vi "My Nonlinear Curve Fit LM bounds.vi"(0 "Y":dbl[](array[numeric]), 1 "f(x,a)":T4, 2 "data":variant, 5 "X":dbl[](array[numeric]), 7 "Weight":dbl[](array[numeric]), 9 "initial parameters":dbl[](array[numeric]), 11 "error in (no error)":errorcluster, 12 "termination":cluster{"max iteration":i32, "tolerance":dbl}={"max iteration"=200, "tolerance"=1e-08}, 13 "parameter bounds":T2, 14 "method":T3 items=["Least Square", "Least Absolute Residual", "Bisquare"]) -> (3 "Fit Aborted?":bool, 4 "best nonlinear fit":dbl[](array[numeric]), 6 "best fit parameters":dbl[](array[numeric]), 8 "covariance":T5, 10 "Fit Statistics":T1, 15 "error out":errorcluster)   [LabVIEW 2019]
uses:
  <vilib>/Analysis/Matrix/Datatypes/RealMatrix.ctl
  <vilib>/gmath/NumericalOptimization/LM model function reference.ctl
  <vilib>/Analysis/6fits.llb/Curve Fitting Criteria.ctl
  Fit Statistics.ctl
  My Fit Stopping Criteria.ctl
  <vilib>/gmath/NumericalOptimization/LM model function.ctl
  <vilib>/gmath/NumericalOptimization/LM_output select.ctl
  Abort Fit Global.vi
  <vilib>/gmath/NI_Gmath.lvlib
  <vilib>/Analysis/NI_AALBase.lvlib
  <vilib>/Analysis/Matrix/NI_Matrix.lvlib
  <vilib>/Analysis/NI_AALPro.lvlib
panel:
  out "Waveform Graph":dbl[](graph)
  in  "Delay (ms)":i32
  in  "Debug":bool
  out "Parameters Chart":dbl[][](graph)
  out "Function & Fit Graph":cluster{"New Coefficients":dbl[]}[](graph)
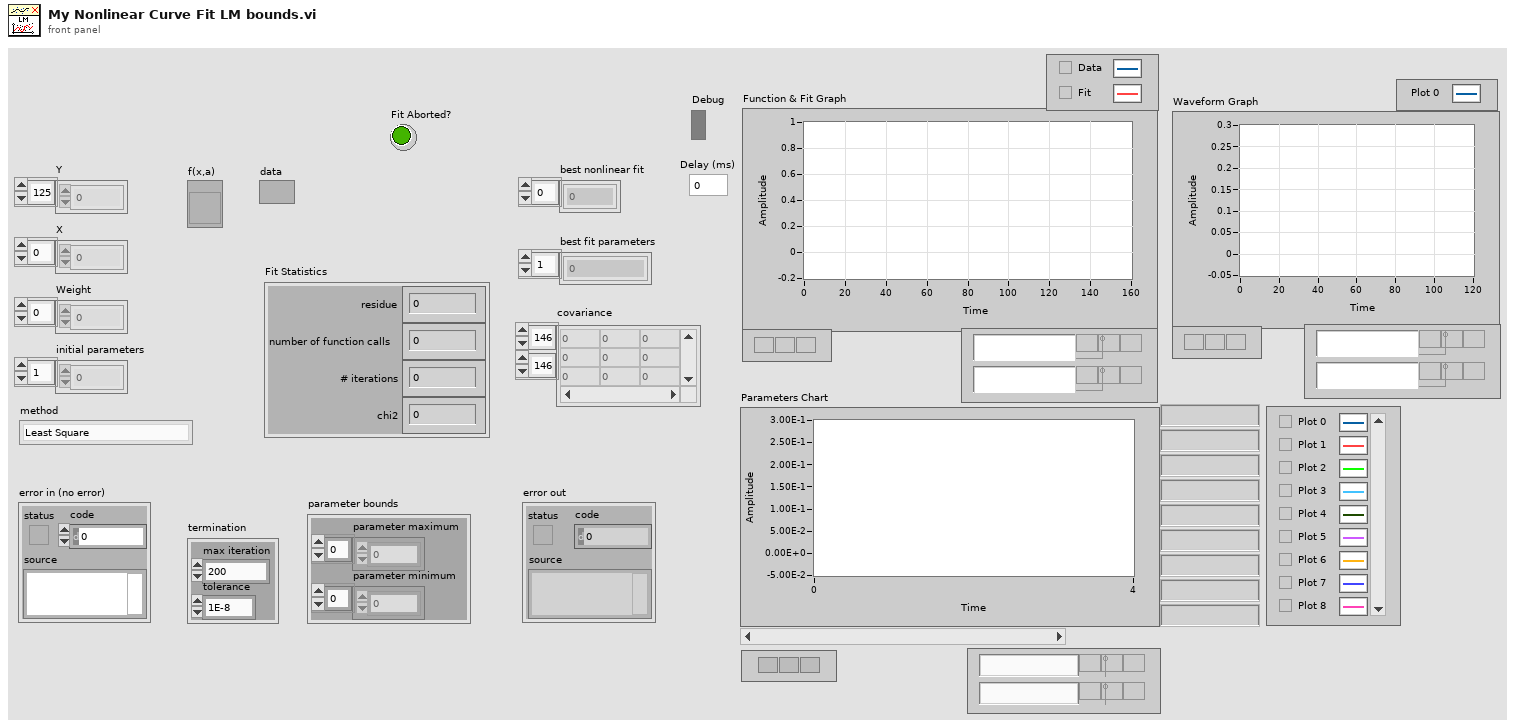
[diagram p1: front panel]
types:
  T1 = typedef "Fit Statistics.ctl" = cluster{"# iterations":i32, "number of function calls":i32, "chi2":dbl, "residue":dbl}
  T2 = cluster{"parameter minimum":dbl[], "parameter maximum":dbl[]}
  T3 = typedef "NI_AALPro.lvlib/Curve Fitting Criteria.ctl" = u16
  T4 = typedef "NI_Gmath.lvlib/LM model function reference.ctl" = refnum<vi>
  T5 = typedef "NI_Matrix.lvlib/RealMatrix.ctl" = dbl[][]
  T6 = typedef "NI_Gmath.lvlib/LM model function.ctl" = cluster{"f(x,a)":T4, "data":variant}
  T7 = typedef "My Fit Stopping Criteria.ctl" = cluster{"function tolerance":dbl, "parameter tolerance":dbl, "max iterations":i32, "max function calls":i32, "gradient tolerance":dbl, "max time (sec)":dbl, "initial tick count":u32, "min lambda":dbl, "max lambda":dbl}
  T8 = typedef "NI_Gmath.lvlib/LM_output select.ctl" = cluster{"model function":bool, "gradient":bool}
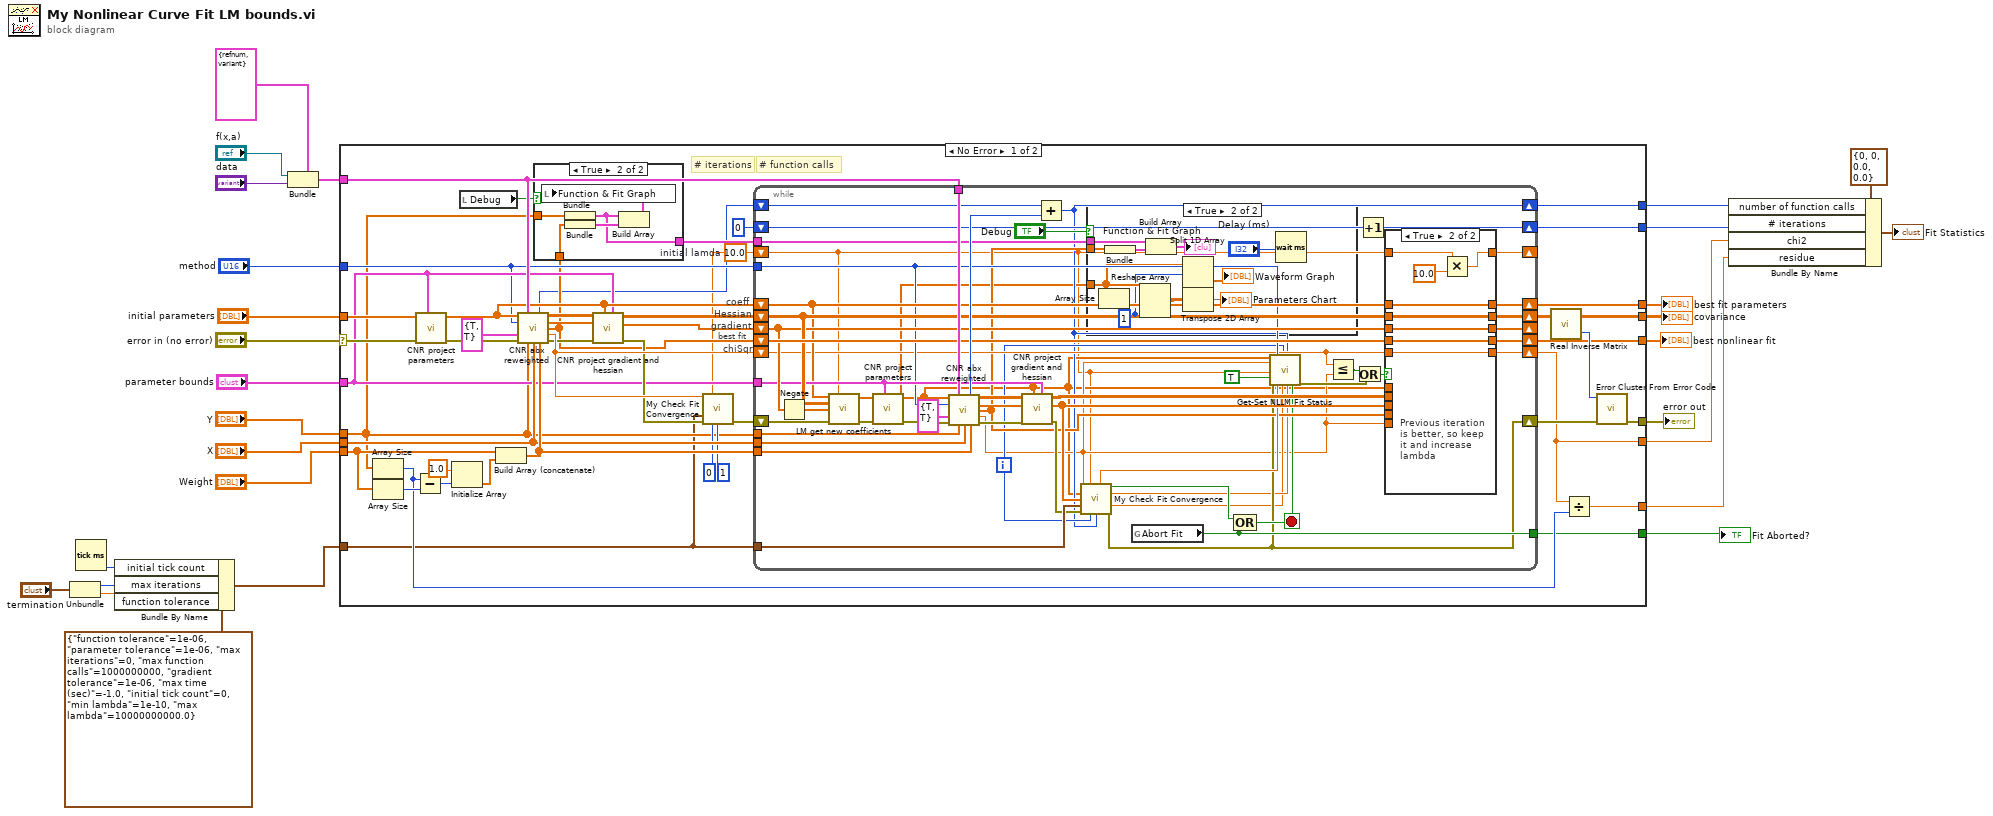
[diagram p0: block diagram]
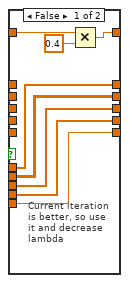
[diagram p4: hidden frame]
diagram:
  n1 = Unbundle("termination") -> ("max iteration"=w17:i32, "tolerance"=w16:dbl)
  n2 = Tick Count (ms)() -> (millisecond timer value=w2:u32)
  n3 = Bundle By Name(cluster=T7 {"function tolerance"=1e-06, "parameter tolerance"=1e-06, "max iterations"=0, "max function calls"=1000000000, "gradient tolerance"=1e-06, "max time (sec)"=-1.0, "initial tick count"=0, "min lambda"=1e-10, "max lambda"=10000000000.0} ("my stopping criteria"), "initial tick count"=w2, "max iterations"=w17, "function tolerance"=w16) -> (w1:T7)
  n4 = Bundle(cluster=T6 {"f(x,a)"=refnum, "data"=variant} ("model function"), "f(x,a)"="f(x,a)", "data"="data") -> (w13:T6)
  n5 = case shown="No Error" "error in (no error)" {
    selector: "error in (no error)" -> [w49 w160]
    tunnel: [w52 _] -> w28
    tunnel: [w73 _] -> w4
    tunnel: "initial parameters" -> [w50 _]
    tunnel: [w60 _] -> w26
    tunnel: [w71 _] -> w25
    tunnel: "Weight" -> [w67 _]
    tunnel: "Y" -> [w37 _]
    tunnel: w1 -> [w30 _]
    tunnel: "X" -> [w61 _]
    tunnel: [w65 w160] -> w21
    tunnel: w13 -> [w62 _]
    tunnel: [w54 _] -> w8
    tunnel: "method" -> [w39 _]
    tunnel: "parameter bounds" -> [w42 _]
    tunnel: [w38 _] -> w9
    tunnel: [w33 _] -> w5
    tunnel: [w31 _] -> w6
    frame No Error {
      w29 = 10.0  # initial lamda
      # "# iterations"
      # "# function calls"
      # "best fit"
      # "chiSqr"
      # "gradient"
      # "Hessian"
      # "coeff"
      n6 = Array Size(array=w37) -> (size(s)=w51:i32)
      n7 = Array Size(array=w67) -> (size(s)=w70:i32)
      n8 = Subtract(x=w51, y=w70) -> (x-y=w69:i32)
      n9 = call <vilib>:"CNR project parameters.vi"("bounds"=w42, "error in"=w49, "parameters"=w50) -> ("error out"=w48:errorcluster, "projected parameters"=w43:dbl[])  [unwired: 7 out]
      n10 = Initialize Array(1.0, w69) -> (w68:dbl[])
      n11 = local read "Debug"() -> (w34:bool)
      n12 = Build Array (concatenate)(w67, w68) -> (w74:dbl[])
      n13 = call <vilib>:"CNR abx reweighted.vi"("parameters"=w43, "model function"=w62, "method"=w39, "output control"=T8 {"model function"=TRUE, "gradient"=TRUE}, "error in (no error)"=w48, "Y"=w37, "X"=w61, "Weight"=w74) -> ("number of function calls"=w32:i32, "Hessian"=w45:T5, "gradient"=w44:dbl[], "best fit"=w35:dbl[], "chiSqr"=w64:dbl, "error out"=w47:errorcluster)  [unwired: 1 in, 1 out]
      n14 = case shown="True" w34 {
        tunnel: w37 -> [_ w79]
        tunnel: [_ w76] -> w36
        tunnel: w35 -> [_ w78]
        frame False {
        }
        frame True {
          n15 = Bundle("Y"=w79) -> (w76:cluster{"Y":dbl[]})  [unwired: 1 in]
          n16 = Bundle("best fit"=w78) -> (w77:cluster{"best fit":dbl[]})  [unwired: 1 in]
          n17 = Build Array(w76, w77) -> (w75:cluster{"best fit":dbl[]}[])
          n18 = local write "Function & Fit Graph"(w75) -> ()
        }
      }
      n19 = call <vilib>:"CNR project gradient and hessian.vi"("bounds"=w42, "projected parameters"=w43, "error in"=w47, "gradient"=w44, "Hessian"=w45) -> ("error out"=w46:errorcluster, "projected gradient"=w40:dbl[], "projected Hessian"=w41:T5)  [unwired: 1 in, 3 out]
      n20 = call "My Check Fit Convergence.vi"("Chi 2"=w64, "Lambda"=w29, "my stopping criteria"=w30, "Error In"=w46, "current iteration"=0, "number of function evaluations"=1) -> ("error out"=w63:errorcluster)  [unwired: 5 in, 4 out]
      n21 = while {
        tunnel: w61 -> [w127]
        tunnel: w37 -> [w95]
        tunnel: w74 -> [w126]
        shift-left: w64 -> [w99]
        shift-right: [w114] -> w33
        shift-left: w40 -> [w120]
        shift-right: [w130] -> _
        shift-left: w41 -> [w121]
        shift-right: [w131] -> w56
        shift-left: w43 -> [w101]
        shift-right: [w115] -> w52
        shift-left: w29 -> [w80]
        shift-right: [w128] -> _
        shift-right: [w86] -> w59
        shift-left: w63 -> [w129]
        tunnel: w62 -> [w125]
        tunnel: w30 -> [w117]
        shift-right: [w88] -> w54
        shift-left: w32 -> [w124]
        shift-right: [w122] -> w60
        shift-left: w35 -> [w123]
        shift-right: [w90] -> w31
        shift-left: 0 -> [w91]
        tunnel: w39 -> [w100]
        tunnel: w42 -> [w107]
        tunnel: [w102] -> w38
        tunnel: w36 -> [w94]
        i -> [w89]
        stop <- w87 stop-if-true
        n22 = Negate(x=w120) -> (-x=w103:dbl[])
        n23 = call <vilib>:"LM get new coefficients.vi"("Coefficients"=w101, "lamda"=w80, "Alpha"=w121, "Beta"=w103, "error in (no error)"=w129) -> ("New Coefficients"=w96:dbl[], "error out"=w113:errorcluster)  [unwired: 9 out]
        n24 = call <vilib>:"CNR project parameters.vi"("bounds"=w107, "error in"=w113, "parameters"=w96) -> ("error out"=w112:errorcluster, "projected parameters"=w81:dbl[])  [unwired: 7 out]
        n25 = call <vilib>:"CNR abx reweighted.vi"("parameters"=w81, "model function"=w125, "method"=w100, "output control"=T8 {"model function"=TRUE, "gradient"=TRUE}, "error in (no error)"=w112, "Y"=w95, "X"=w127, "Weight"=w126) -> ("number of function calls"=w132:i32, "Hessian"=w106:T5, "gradient"=w109:dbl[], "best fit"=w92:dbl[], "chiSqr"=w82:dbl, "error out"=w111:errorcluster)  [unwired: 1 in, 1 out]
        n26 = call <vilib>:"CNR project gradient and hessian.vi"("bounds"=w107, "projected parameters"=w81, "error in"=w111, "gradient"=w109, "Hessian"=w106) -> ("error out"=w110:errorcluster, "projected gradient"=w108:dbl[], "projected Hessian"=w105:T5)  [unwired: 1 in, 3 out]
        n27 = Add(x=w124, y=w132) -> (x+y=w88:i32)
        n28 = call "My Check Fit Convergence.vi"("Chi 2"=w82, "Lambda"=w80, "Parameters"=w81, "gradient"=w108, "my stopping criteria"=w117, "Error In"=w110, "current iteration"=w89, "number of function evaluations"=w88) -> ("|Delta Chi 2|/Chi 2"=w97:dbl, "stop?"=w116:bool, "|Delta Chi 2|"=w84:dbl, "Max |Delta a| /|a|"=w83:dbl, "error out"=w86:errorcluster)  [unwired: 3 in]
        n29 = case shown="True" "Debug" {
          tunnel: w81 -> [_ w135]
          tunnel: w94 -> [_ w143]
          tunnel: w92 -> [_ w140]
          frame False {
          }
          frame True {
            w133 = 1 ("dimension size")
            n30 = Array Size(array=w135) -> (size(s)=w139:i32)
            n31 = Bundle("best fit"=w140) -> (w142:cluster{"best fit":dbl[]})  [unwired: 1 in]
            n32 = Reshape Array(w135, w139, w133) -> (w138:dbl[][])
            n33 = Build Array(w143, w142) -> (→"Function & Fit Graph":cluster{"best fit":dbl[]}[])
            n34 = Split 1D Array(array=w135, index=w133) -> (second subarray=→"Waveform Graph":dbl[])  [unwired: 1 out]
            n35 = Transpose 2D Array(2D array=w138) -> (transposed array=→"Parameters Chart":dbl[][])
            n36 = Wait (ms)(milliseconds to wait="Delay (ms)") -> ()  [unwired: 1 out]
          }
        }
        n37 = global read "Abort Fit Global.vi" "Abort Fit"() -> (w102:bool)
        n38 = Compound Arithmetic op=OR(w116, w102) -> (w87:bool)
        n39 = call "Get-Set NLLM Fit Status.vi"("Fit Parameters"=w81, "chiSqr"=w82, "Lambda"=w80, "Get(F)/Set"=TRUE, "Error In"=w86, "method"=w100, "|Delta Chi 2|/Chi 2"=w97, "# Iterations"=w89, "Max |Delta a| /|a|"=w83, "# Function Calls"=w88, "|Delta Chi 2|"=w84, "Done"=w87) -> ("Error Out"=w85:errorcluster)  [unwired: 6 in, 1 out]
        n40 = Less Or Equal?(x=w99, y=w82) -> (x <= y?=w119:bool)
        n41 = Or(x=w119, y=w85) -> (x .or. y?=w118:bool)
        n42 = Increment(x=w91) -> (x+1=w90:i32)
        n43 = case shown="True" w118 {
          tunnel: [w150 w159] -> w131
          tunnel: w121 -> [_ w159]
          tunnel: [w149 w158] -> w130
          tunnel: w81 -> [w146 _]
          tunnel: w120 -> [_ w158]
          tunnel: w101 -> [_ w157]
          tunnel: [w146 w157] -> w115
          tunnel: [w151 w155] -> w128
          tunnel: w99 -> [_ w156]
          tunnel: w82 -> [w147 _]
          tunnel: [w147 w156] -> w114
          tunnel: w80 -> [w145 w153]
          tunnel: w105 -> [w150 _]
          tunnel: w108 -> [w149 _]
          tunnel: w123 -> [_ w154]
          tunnel: w92 -> [w148 _]
          tunnel: [w148 w154] -> w122
          frame False {
            # "Current iteration\nis better, so use\nit and decrease \nlambda"
            n44 = Multiply(x=w145, y=0.4) -> (x*y=w151:dbl)
          }
          frame True {
            # "Previous iteration\nis better, so keep\nit and increase \nlambda"
            n45 = Multiply(x=w153, y=10.0) -> (x*y=w155:dbl)
          }
        }
      }
      n46 = call <vilib>:"Real Inverse Matrix.vi"("Input Matrix"=w56) -> ("error"=w66:i32, "Inverse Matrix"=w71:T5)  [unwired: 1 in]
      n47 = Divide(x=w33, y=w51) -> (x/y=w73:dbl)
      n48 = call <vilib>:"Error Cluster From Error Code.vi"("error in (no error)"=w59, "error code (0)"=w66) -> ("error out"=w65:errorcluster)  [unwired: 1 in, 6 out]
    }
    frame Error {
    }
  }
  "best fit parameters" <- w28
  "best nonlinear fit" <- w26
  "error out" <- w21
  "covariance" <- w25
  "Fit Aborted?" <- w9
  n49 = Bundle By Name(cluster=T1 {"# iterations"=0, "number of function calls"=0, "chi2"=0.0, "residue"=0.0} ("Fit Statistics"), "number of function calls"=w8, "# iterations"=w6, "chi2"=w5, "residue"=w4) -> (→"Fit Statistics":T1)
